vi "Untitled 2.vi"() -> ()   [LabVIEW 2017]
panel:
  out "Array 3":i32[](array[numeric])
  out "Array 2":i32[](array[numeric])
  out "Elapsed Time":dbl
  out "Boolean":bool
  in  "stop":bool
  in  "Array":bool[](array[boolean])
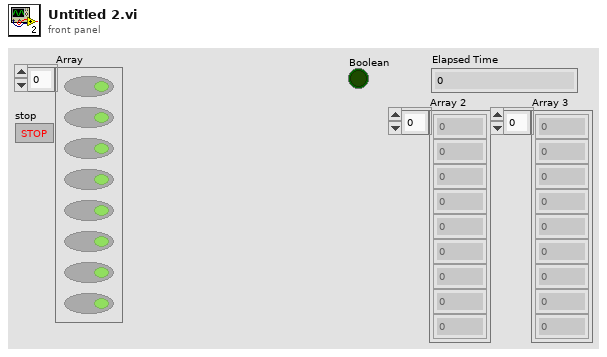
[diagram p1: front panel]
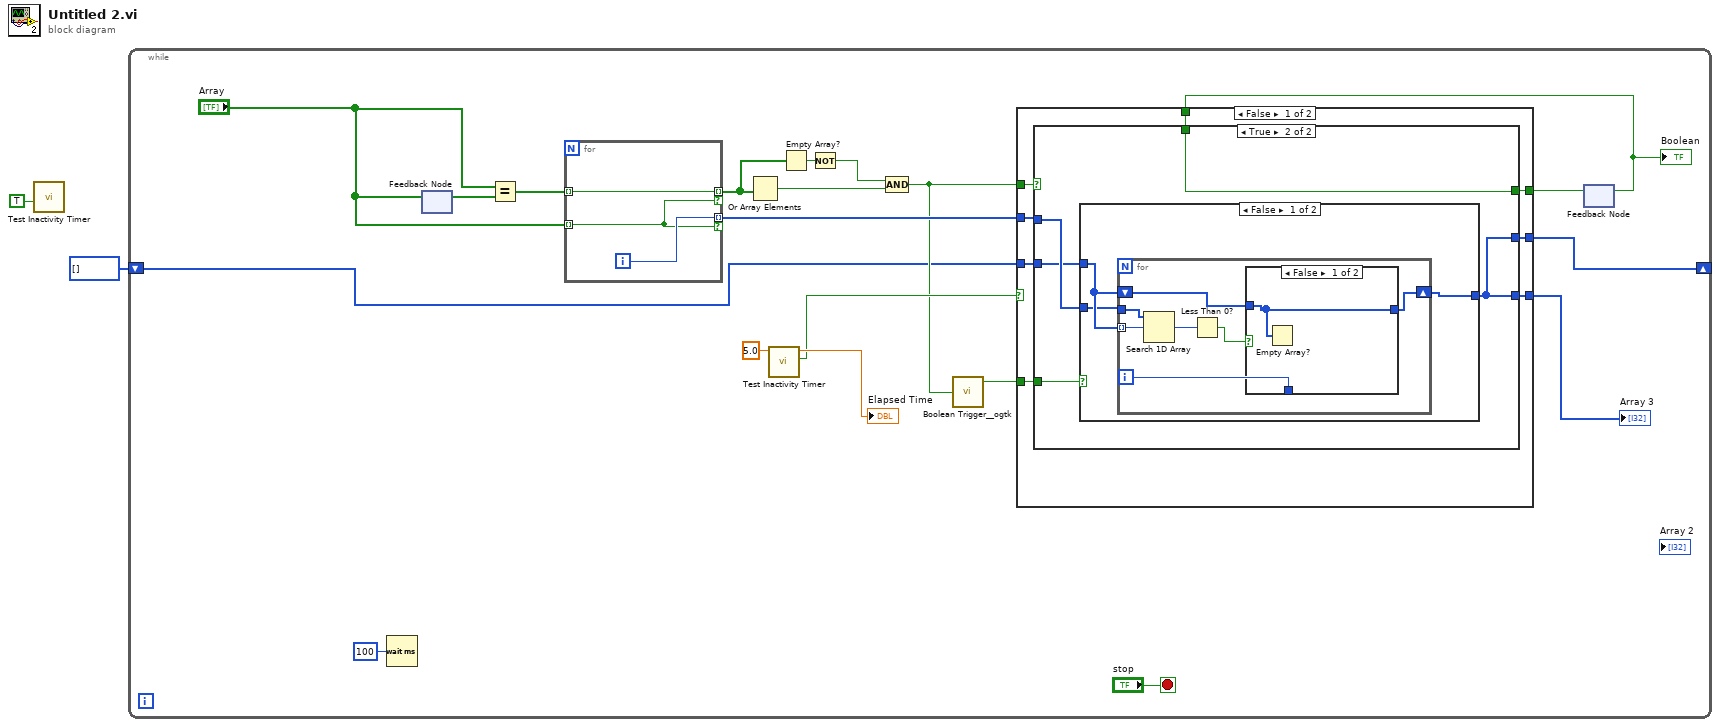
[diagram p0: block diagram]
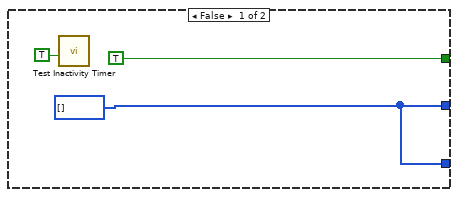
[diagram p2: hidden frame]
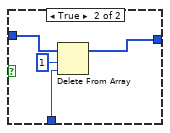
[diagram p3: hidden frame]
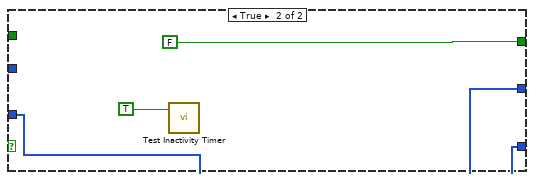
[diagram p5: hidden frame]
diagram:
  n1 = call "Test Inactivity Timer.vi"("Reset"=TRUE) -> ()  [unwired: 8 in, 3 out]
  n2 = while {
    shift-right: [w15] -> _
    shift-left: i32[] [] -> [w3]
    stop <- "stop" stop-if-true
    n3 = Wait (ms)(milliseconds to wait=u32 100) -> ()  [unwired: 1 out]
    n4 = feedback #1() -> (w14:bool[])  [unwired: 1 in]
    n5 = feedback-in #1("Array") -> ()
    n6 = Equal?(x="Array", y=w14) -> (x = y?=w12:bool[])
    n7 = for {
      tunnel: [w58] -> w11 mode=indexing if=w59
      tunnel: w12 -> [w58] mode=indexing
      tunnel: [w60] -> w8 mode=indexing if=w59
      tunnel: "Array" -> [w59] mode=indexing
      i -> [w60]
    }
    n8 = Or Array Elements(Boolean array=w11) -> (logical OR=w13:bool)
    n9 = call "Test Inactivity Timer.vi"("Target Time"=5.0) -> ("Time Elapsed"=w7:bool, "Elapsed Time"=→"Elapsed Time":dbl)  [unwired: 8 in, 1 out]
    n10 = Empty Array?(array=w11) -> (empty?=w10:bool)
    n11 = Not(x=w10) -> (.not. x?=w9:bool)
    n12 = Compound Arithmetic op=AND(w9, w13) -> (w6:bool)
    n13 = call <userlib>:"Boolean Trigger__ogtk.vi"("Boolean Input"=w6) -> ("Rising Edge"=w5:bool)  [unwired: 1 in, 1 out]
    n14 = feedback #2() -> (w16:bool)  [unwired: 1 in]
    "Boolean" <- w16
    n15 = case shown="False" w7 {
      tunnel: [w30 FALSE ("Boolean")] -> w17
      tunnel: w16 -> [w29 _]
      tunnel: [w28 w55] -> w15
      tunnel: w6 -> [w27 _]
      tunnel: w8 -> [w26 _]
      tunnel: w5 -> [w25 _]
      tunnel: [w24 w55] -> w4
      tunnel: w3 -> [w23 w55]
      frame False {
        n16 = case shown="True" w27 {
          tunnel: [TRUE ("Boolean") w38] -> w30
          tunnel: w29 -> [_ w38]
          tunnel: w26 -> [_ w36]
          tunnel: [w31 w35] -> w28
          tunnel: w25 -> [_ w37]
          tunnel: [w31 w35] -> w24
          tunnel: w23 -> [_ w34]
          frame False {
            w31 = i32[] []
            n17 = call "Test Inactivity Timer.vi"("Reset"=TRUE) -> ()  [unwired: 8 in, 3 out]
          }
          frame True {
            n18 = case shown="False" w37 {
              tunnel: [w40 w54] -> w35
              tunnel: w36 -> [w39 w54]
              tunnel: w34 -> [w41 _]
              frame False {
                n19 = for {
                  tunnel: w41 -> [w48] mode=indexing
                  tunnel: w39 -> [w47]
                  shift-right: [w44] -> w40
                  shift-left: w41 -> [w42]
                  i -> [w43]
                  n20 = Search 1D Array(1D array=w47, element=w48) -> (index of element=w45:i32)  [unwired: 1 in]
                  n21 = Less Than 0?(x=w45) -> (x < 0?=w46:bool)
                  n22 = case shown="False" w46 {
                    tunnel: w42 -> [w49 w53]
                    tunnel: w43 -> [_ w51]
                    tunnel: [w49 w50] -> w44
                    frame False {
                      n23 = Empty Array?(array=w49) -> ()  [unwired: 1 out]
                    }
                    frame True {
                      n24 = Delete From Array(array=w53, length=1, index=w51) -> (array with subset deleted=w50:i32[])  [unwired: 1 out]
                    }
                  }
                }
              }
              frame True {
              }
            }
          }
        }
      }
      frame True {
        n25 = call "Test Inactivity Timer.vi"("Reset"=TRUE) -> ()  [unwired: 8 in, 3 out]
      }
    }
    "Array 3" <- w4
    n26 = feedback-in #2(w17) -> ()
  }
